vi "Label Targets_Custom.vi"(8 "Score Threshold":dbl=75.0, 9 "Annotate":bool=TRUE, 10 "Targets":T2(array[cluster]), 11 "Image in":T1) -> (3 "Image out":T1)   [LabVIEW 2015]
doc: "Draw text scores near or on the particle. Scores above the limit are green and underlined."
uses:
  <vilib>/vision/Image Controls.llb/IMAQ Image.ctl
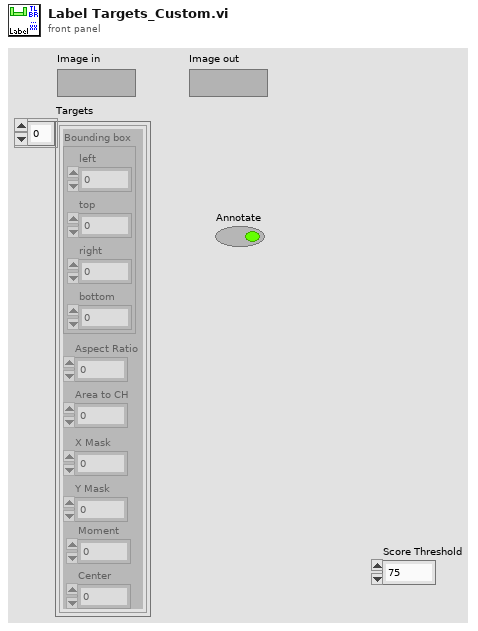
[diagram p1: front panel]
types:
  T1 = typedef "IMAQ Image.ctl" = refnum<image>
  T2 = cluster{"Bounding box":cluster{"left":dbl, "top":dbl, "right":dbl, "bottom":dbl}, "Aspect Ratio":dbl, "Area to CH":dbl, "X Mask":dbl, "Y Mask":dbl, "Moment":dbl, "Center":dbl}[]
  T3 = cluster{"Desired Font (Application)":enum16{"User-specified Font", "Application Font", "System Font", "Dialog Font"}, "[User-specified Font]":cluster{"Font Name":string, "Size":i16, "Strikeout?":bool, "Italic?":bool, "Underline?":bool, "Outline?":bool, "Shadow?":bool, "Bold?":bool, "Rotation Angle":dbl}, "Horizontal Alignment":i16, "Vertical Alignment":i16}
  T4 = cluster{"left":dbl, "top":dbl, "right":dbl, "bottom":dbl}
  T5 = cluster{"Aspect Ratio":dbl, "Area to CH":dbl, "X Mask":dbl, "Y Mask":dbl, "Moment":dbl}
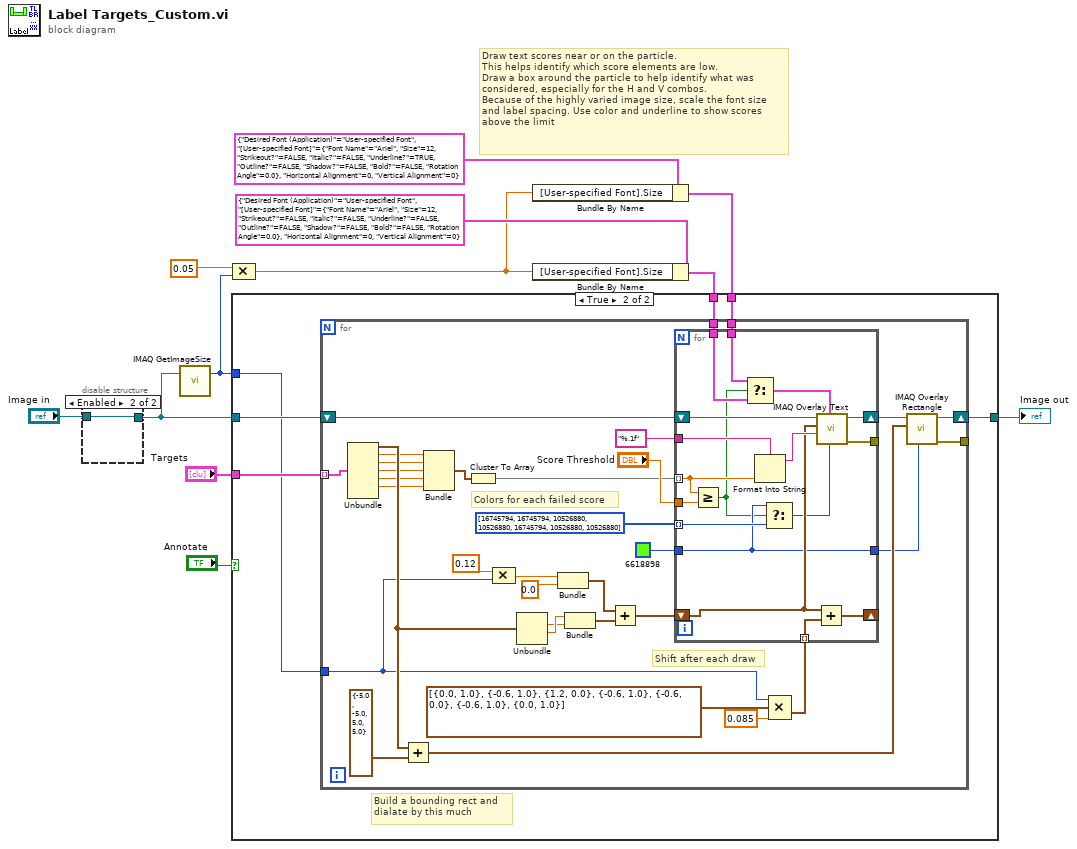
[diagram p0: block diagram]
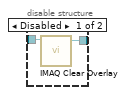
[diagram p2: hidden frame]
diagram:
  # "Draw text scores near or on the particle.\nThis helps identify which score elements are low.\nDraw a box around the particle to help identify what was\nconsidered, especially for the H and V combos.\nBecause of the highly varied image size, scale the font size\nand label spacing. Use color and underline to show scores\nabove the limit"
  n1 = disable-structure shown="Enabled" {
    disable-tunnel: "Image in" -> [w14 w15]
    disable-tunnel: [w13 w15] -> w4
    frame Disabled {
      n2 = call "IMAQ Clear Overlay"("Image"=w14) -> ("Image Out"=w13:T1)  [unwired: 2 in, 8 out]
    }
    frame Enabled {
    }
  }
  n3 = call "IMAQ GetImageSize"("Image"=w4) -> ("Y Resolution"=w3:i32)  [unwired: 3 in, 2 out]
  n4 = Compound Arithmetic op=MULTIPLY(0.05, w3) -> (w2:dbl)
  n5 = Bundle By Name(cluster=T3 {"Desired Font (Application)"=enum."User-specified Font", "[User-specified Font]"={"Font Name"="Ariel", "Size"=12, "Strikeout?"=FALSE, "Italic?"=FALSE, "Underline?"=TRUE, "Outline?"=FALSE, "Shadow?"=FALSE, "Bold?"=FALSE, "Rotation Angle"=0.0}, "Horizontal Alignment"=0, "Vertical Alignment"=0} ("Font, Size & Style"), "[User-specified Font].Size"=w2) -> (w5:T3)
  n6 = Bundle By Name(cluster=T3 {"Desired Font (Application)"=enum."User-specified Font", "[User-specified Font]"={"Font Name"="Ariel", "Size"=12, "Strikeout?"=FALSE, "Italic?"=FALSE, "Underline?"=FALSE, "Outline?"=FALSE, "Shadow?"=FALSE, "Bold?"=FALSE, "Rotation Angle"=0.0}, "Horizontal Alignment"=0, "Vertical Alignment"=0} ("Font, Size & Style"), "[User-specified Font].Size"=w2) -> (w6:T3)
  n7 = case shown="True" "Annotate" {
    tunnel: [w16 w22] -> w12
    tunnel: "Targets" -> [_ w21]
    tunnel: w4 -> [w16 w20]
    tunnel: w5 -> [_ w19]
    tunnel: w6 -> [_ w18]
    tunnel: w3 -> [_ w17]
    frame False {
    }
    frame True {
      # "Build a bounding rect and\ndialate by this much"
      n8 = for {
        tunnel: w21 -> [w50] mode=indexing
        shift-right: [w51] -> w22
        shift-left: w20 -> [w56]
        tunnel: w17 -> [w26]
        tunnel: w19 -> [w31]
        tunnel: w18 -> [w30]
        tunnel: [w23] -> _
        # "Colors for each failed score"
        # "Shift after each draw"
        n9 = Unbundle(w50) -> ("Bounding box"=w44:T4, "Aspect Ratio"=w42:dbl, "Area to CH"=w41:dbl, "X Mask"=w39:dbl, "Y Mask"=w40:dbl, "Moment"=w24:dbl)  [unwired: 1 out]
        n10 = Add(x=w44, y=cluster{dbl, dbl, dbl, dbl} {-5.0, -5.0, 5.0, 5.0} ("output cluster")) -> (x+y=w46:cluster{dbl, dbl, dbl, dbl})
        n11 = Bundle("Aspect Ratio"=w42, "Area to CH"=w41, "X Mask"=w39, "Y Mask"=w40, "Moment"=w24) -> (w53:T5)  [unwired: 1 in]
        n12 = Cluster To Array(cluster=w53) -> (array=w43:dbl[])
        n13 = Compound Arithmetic op=MULTIPLY(0.12, w26) -> (w27:dbl)
        n14 = Unbundle(w44) -> ("top"=w48:dbl, "right"=w49:dbl)  [unwired: 2 out]
        n15 = Bundle(w27, 0.0) -> (w29:cluster{dbl, dbl})  [unwired: 1 in]
        n16 = Bundle("right"=w49, "top"=w48) -> (w47:cluster{"right":dbl, "top":dbl})  [unwired: 1 in]
        n17 = Add(x=w29, y=w47) -> (x+y=w55:cluster{dbl, dbl})
        n18 = Compound Arithmetic op=MULTIPLY(w26, cluster{dbl, dbl}[] [{0.0, 1.0}, {-0.6, 1.0}, {1.2, 0.0}, {-0.6, 1.0}, {-0.6, 0.0}, {-0.6, 1.0}, {0.0, 1.0}], 0.085) -> (w35:cluster{dbl, dbl}[])
        n19 = for {
          tunnel: w43 -> [w67] mode=indexing
          shift-right: [w70] -> _
          shift-left: w55 -> [w69]
          shift-right: [w71] -> w52
          shift-left: w56 -> [w72]
          tunnel: u32[] [16745794, 16745794, 10526880, 10526880, 16745794, 10526880, 10526880] -> [w68] mode=indexing
          tunnel: "Score Threshold" -> [w66]
          tunnel: w35 -> [w64] mode=indexing
          tunnel: "%.1f" ("format string") -> [w63]
          tunnel: u32 6618898 ("Color") -> [w62]
          tunnel: [w62] -> w37
          tunnel: w31 -> [w61]
          tunnel: w30 -> [w60]
          tunnel: [w57] -> _
          n20 = Greater Or Equal?(x=w67, y=w66) -> (x >= y?=w59:bool)
          n21 = Select(t=w61, s=w59, f=w60) -> (s? t:f=w58:T3)
          n22 = Format Into String(format string=w63, w67) -> (resulting string=w73:string)  [unwired: 2 in, 1 out]
          n23 = Select(t=w62, s=w59, f=w68) -> (s? t:f=w65:u32)
          n24 = Add(x=w64, y=w69) -> (x+y=w70:cluster{dbl, dbl})
          n25 = call "IMAQ Overlay Text"("Text Color (black)"=w65, "Font, Size & Style"=w58, "String"=w73, "Origin"=w69, "Image"=w72) -> ("error out"=w57:errorcluster, "Image Out"=w71:T1)  [unwired: 5 in]
        }
        n26 = call "IMAQ Overlay Rectangle"("Color"=w37, "Rectangle"=w46, "Image"=w52) -> ("error out"=w23:errorcluster, "Image Out"=w51:T1)  [unwired: 7 in]
      }
    }
  }
  "Image out" <- w12
